vi "Get DI Status - All.vi"(0 "reference in":refnum<class "DI.lvclass">, 5 "error in (no error)":errorcluster) -> (14 "reference out":refnum<class "DI.lvclass">, 16 "All DI Status":bool[](array[boolean]), 19 "error out":errorcluster)   [LabVIEW 2017, in "DI.lvclass"]
uses:
  DI.lvclass
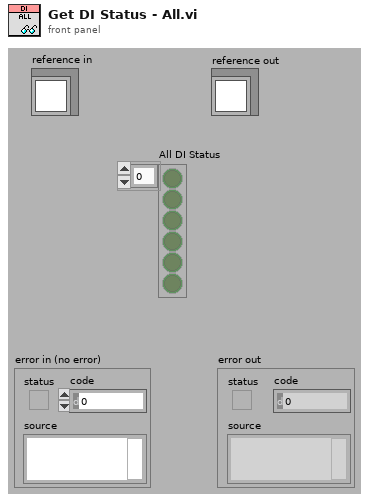
[diagram p1: front panel]
types:
  T1 = typedef "DI.lvclass/ObjectAttributes.ctl" = cluster{"DI Task":refnum<k21>, "DI Status":bool[], "DI Module Names (NI-Max Name)":string[], "Number of Channels Per DI Module":i32[], "Number of DI Modules":u32, "Number of Total DI Channels":u32, "DI On/Off Status":bool, "DO VI Reference":refnum<vi>}
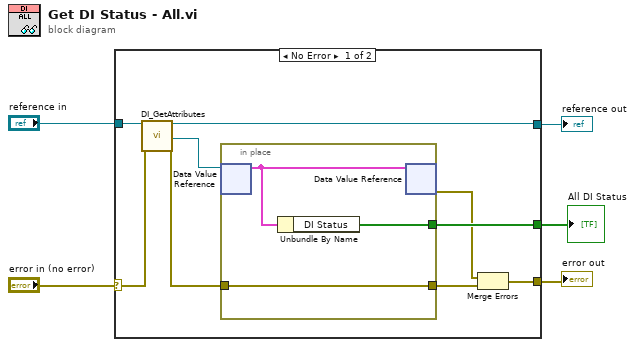
[diagram p0: block diagram]
diagram:
  n1 = case shown="No Error" "error in (no error)" {
    selector: "error in (no error)" -> [w13 w19]
    tunnel: [w11 w19] -> w4
    tunnel: [w12 w18] -> w2
    tunnel: "reference in" -> [w14 w18]
    tunnel: [w7 _] -> w1
    frame No Error {
      n2 = call "DI_GetAttributes.vi"("reference in"=w14, "error in (no error)"=w13) -> ("reference out"=w12:refnum<class "DI.lvclass">, "DataRef"=w10:refnum<data-value>, "error out"=w9:errorcluster)  [unwired: 14 in, 1 out]
      n3 = in-place {
        in-place-border: w9 -> [w17]
        in-place-border: [w17] -> w8
        in-place-border: [w15] -> w7
        n4 = in-place-dvr #1(w10) -> (w16:T1)  [unwired: 1 out]
        n5 = Unbundle By Name(w16) -> ("DI Status"=w15:bool[])
        n6 = in-place-dvr #1(w16) -> (w6:errorcluster)  [unwired: 1 out]
      }
      n7 = Merge Errors(w6, w8) -> (w11:errorcluster)
    }
    frame Error {
    }
  }
  "error out" <- w4
  "reference out" <- w2
  "All DI Status" <- w1
